vi "Return FPGA Setup Data.vi"(6 "wait for reply (T)":bool=TRUE, 8 "error in (no error)":errorcluster, 10 "Reload":bool) -> (0 "error out":errorcluster, 1 "timed out?":bool, 2 "Reply Payload":T1={"Version String"="", "FPGA Setup Parameters"={"FPGA Timing Constraints"={"frame.length Min"=530, "frame.ST_OFF Min"=15, "frame.ST_ON Min"=8, "frame.first data idx"=14, "frame.integ Offset"=6, "frame.integ Delay"=3, "frame.ad_latch Delay"=11, "frame.trig time Max"=0}, "FPGA Timing Ctrl"={"trig.time"=220, "integ.count 1"=400, "integ.count 2"=350, "encdr.latch ctrl"=1, "pixel.read count"=512, "clock.select"=2, "ad.clock offset"=16, "data.control reg"=2}, "FPGA Laser Config"={"laser.gain"=10, "laser.threshold Low"=1400, "laser.threshold High"=1900, "laser.dac init"=912, "laser.dac Min"=800, "laser.dac Max"=4000, "laser.config reg"=3}, "FPGA Peak Proc Cfg"={"PD.threshold"=0, "PD.width detect Min"=0, "PD.sensor pixels"=512, "PD.config reg"=23}, "FPGA SPI Cfg"={"SPI Divide Value"=1, "SPI config reg"=1}}, "Return FPGA Setup Data_error"={"status"=FALSE, "code"=0, "source"=""}} {"FPGA Setup Parameters"."FPGA SPI Cfg"."SPI config reg" format="%03b"; "FPGA Setup Parameters"."FPGA Peak Proc Cfg"."PD.config reg" format="%05b"; "FPGA Setup Parameters"."FPGA Laser Config"."laser.config reg" format="%02b"; "FPGA Setup Parameters"."FPGA Timing Ctrl"."data.control reg" format="%03b"; "FPGA Setup Parameters"."FPGA Timing Constraints"."frame.trig time Max" format="%0.0f"})   [LabVIEW 2015, in "Tool Module.lvlib"]
doc: "Returns local copy of FPGA setup data from Tool Module.\n_____\nCreated using Delacor QMH Event Scripter 4.2.1.88."
uses:
  Tool Module.lvlib
  Return FPGA Setup Data (Reply Payload)--cluster.ctl
  Tool Typedefs/_FPGA Setup Params Cluster--typedef.ctl
  Tool Typedefs/_FPGA Timing Constraints Cluster--typedef.ctl
  Tool Typedefs/_FPGA Timing Ctrl Cluster--typedef.ctl
  Tool Typedefs/_FPGA Laser Config Cluster--typedef.ctl
  Tool Typedefs/_FPGA Peak Proc Cfg Cluster--typedef.ctl
  Tool Typedefs/_FPGA SPI Cfg Cluster--typedef.ctl
  Return FPGA Setup Data Argument--cluster.ctl
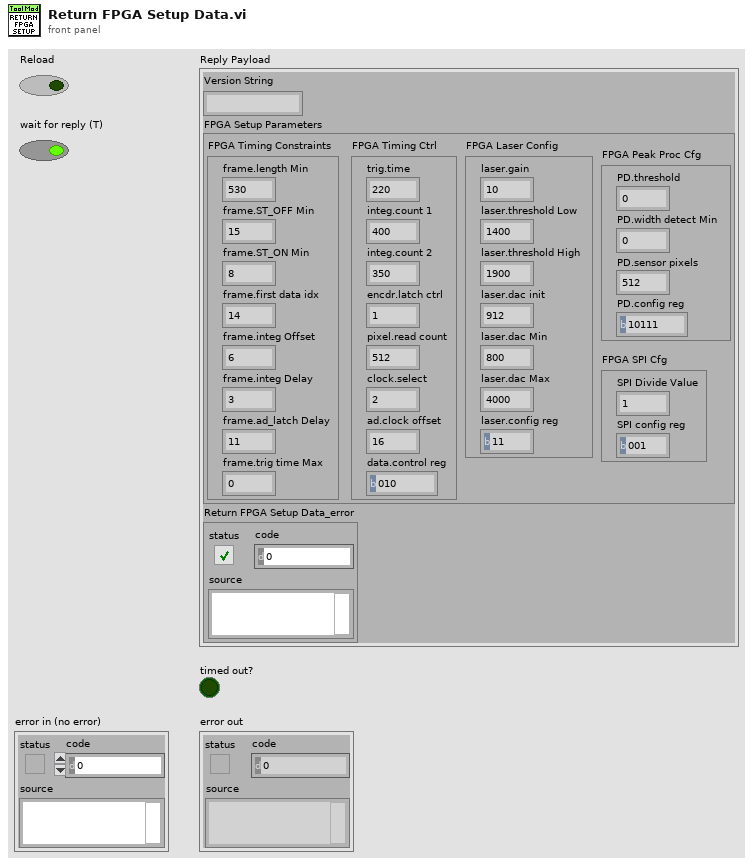
[diagram p1: front panel]
types:
  T1 = typedef "Tool Module.lvlib/Return FPGA Setup Data (Reply Payload)--cluster.ctl" = cluster{"Version String":string, "FPGA Setup Parameters":T2, "Return FPGA Setup Data_error":errorcluster}
  T2 = typedef "_FPGA Setup Params Cluster--typedef.ctl" = cluster{"FPGA Timing Constraints":T3, "FPGA Timing Ctrl":T4, "FPGA Laser Config":T5, "FPGA Peak Proc Cfg":T6, "FPGA SPI Cfg":T7}
  T3 = typedef "_FPGA Timing Constraints Cluster--typedef.ctl" = cluster{"frame.length Min":u16, "frame.ST_OFF Min":u16, "frame.ST_ON Min":u16, "frame.first data idx":u16, "frame.integ Offset":u16, "frame.integ Delay":u16, "frame.ad_latch Delay":u16, "frame.trig time Max":u32}
  T4 = typedef "_FPGA Timing Ctrl Cluster--typedef.ctl" = cluster{"trig.time":u32, "integ.count 1":u32, "integ.count 2":u32, "encdr.latch ctrl":u32, "pixel.read count":u16, "clock.select":u16, "ad.clock offset":u16, "data.control reg":u16}
  T5 = typedef "_FPGA Laser Config Cluster--typedef.ctl" = cluster{"laser.gain":i16, "laser.threshold Low":u16, "laser.threshold High":u16, "laser.dac init":u16, "laser.dac Min":u16, "laser.dac Max":u16, "laser.config reg":u16}
  T6 = typedef "_FPGA Peak Proc Cfg Cluster--typedef.ctl" = cluster{"PD.threshold":u16, "PD.width detect Min":u8, "PD.sensor pixels":u16, "PD.config reg":u16}
  T7 = typedef "_FPGA SPI Cfg Cluster--typedef.ctl" = cluster{"SPI Divide Value":u8, "SPI config reg":u16}
  T8 = typedef "Tool Module.lvlib/Return FPGA Setup Data Argument--cluster.ctl" = cluster{"Reload":bool, "Wait Notifier":refnum<notifier>, "wait for reply":bool}
  T9 = typedef "Tool Module.lvlib/Request Events--cluster.ctl" = cluster{"Stop Module":refnum<user-event>, "Show Panel":refnum<user-event>, "Hide Panel":refnum<user-event>, "Get Module Execution Status":refnum<user-event>, "Show Diagram":refnum<user-event>, "Test Trig 2":refnum<user-event>, "GOTO":refnum<user-event>, "Start Inspect":refnum<user-event>, "CONNECT":refnum<user-event>, "Get All Inspect Data":refnum<user-event>, "Get Inspection Limits":refnum<user-event>, "Set Inspection Limits":refnum<user-event>, "Update Status":refnum<user-event>, "Start Data Monitor":refnum<user-event>, "Get FPGA Setup Params":refnum<user-event>, "Set FPGA Setup Params":refnum<user-event>, "Set Tool Config":refnum<user-event>, "Get Tool Config":refnum<user-event>, "Set Integration Count":refnum<user-event>, "Set Laser Params":refnum<user-event>, "Get Mtrl Ctrl Reg":refnum<user-event>, "Commit Ctrl Reg":refnum<user-event>, "Set Event Logger":refnum<user-event>, "Write to File":refnum<user-event>, "Read from File":refnum<user-event>, "Set Device Temp Thresholds":refnum<user-event>, "Get Cycle Count":refnum<user-event>, "Return FPGA Setup Data":refnum<user-event>, "Update FPGA Setup Data":refnum<user-event>}
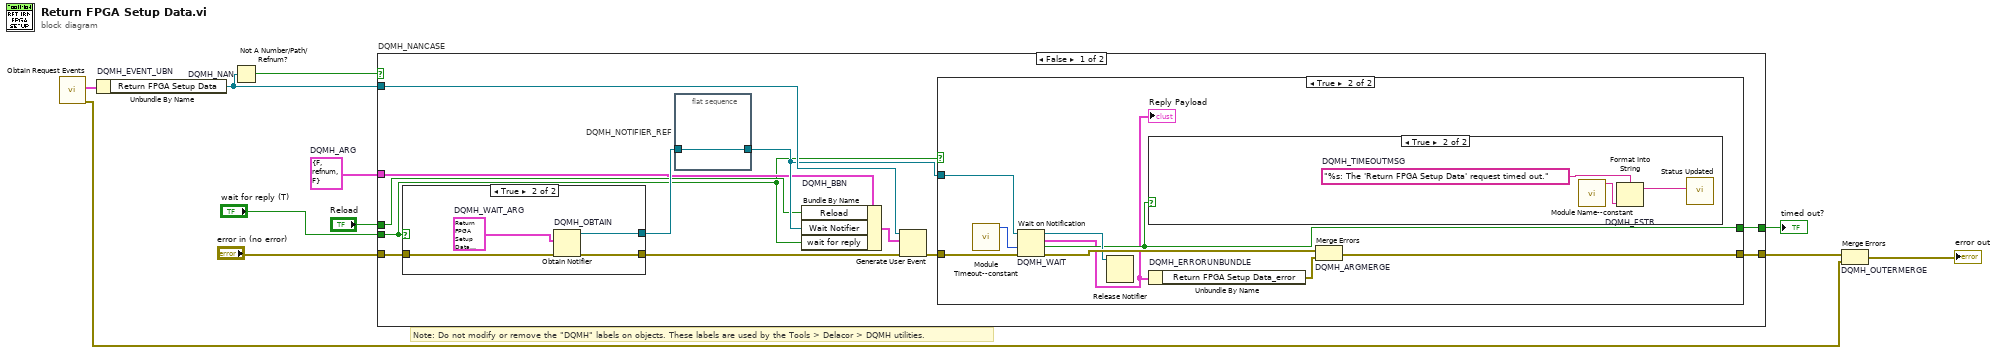
[diagram p0: block diagram]
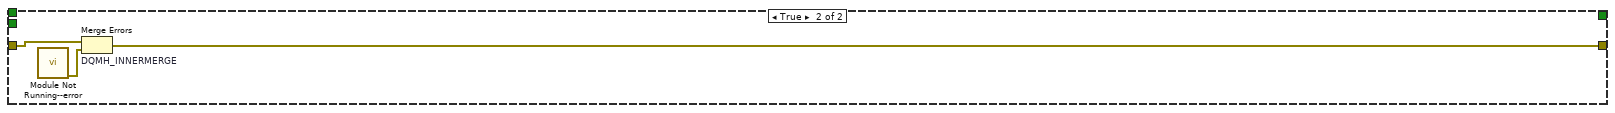
[diagram p5: hidden frame]
diagram:
  w5 = T8 {"Reload"=FALSE, "Wait Notifier"=refnum, "wait for reply"=FALSE}  # DQMH_ARG
  # "Note: Do not modify or remove the \"DQMH\" labels on objects. These labels are used by the Tools > Delacor > DQMH utilities."
  n1 = call "Obtain Request Events.vi"() -> ("error out"=w2:errorcluster, "Tool Module Request Events"=w1:T9)  [unwired: 10 in]
  n2 = Unbundle By Name "DQMH_EVENT_UBN"(w1) -> ("Return FPGA Setup Data"=w9:refnum<user-event>)
  n3 = Not A Number/Path/Refnum? "DQMH_NAN"(number/path/refnum=w9) -> (NaN/Path/Refnum?=w8:bool)
  n4 = case "DQMH_NANCASE" shown="False" w8 {
    tunnel: "error in (no error)" -> [w23 w45]
    tunnel: w9 -> [w21 _]
    tunnel: [w18 w44] -> w6
    tunnel: [w19 _] -> w7
    tunnel: w5 -> [w14 _]
    tunnel: "Reload" -> [w13 _]
    tunnel: "wait for reply (T)" -> [w12 _]
    frame False {
      n5 = case shown="True" w12 {
        tunnel: w23 -> [w38 w42]
        tunnel: [w38 w41] -> w20
        tunnel: [_ w39] -> w16
        frame False {
        }
        frame True {
          w40 = T1 {"Version String"="", "FPGA Setup Parameters"={"FPGA Timing Constraints"={"frame.length Min"=530, "frame.ST_OFF Min"=15, "frame.ST_ON Min"=8, "frame.first data idx"=14, "frame.integ Offset"=6, "frame.integ Delay"=3, "frame.ad_latch Delay"=11, "frame.trig time Max"=0}, "FPGA Timing Ctrl"={"trig.time"=220, "integ.count 1"=400, "integ.count 2"=350, "encdr.latch ctrl"=1, "pixel.read count"=512, "clock.select"=2, "ad.clock offset"=16, "data.control reg"=2}, "FPGA Laser Config"={"laser.gain"=10, "laser.threshold Low"=1400, "laser.threshold High"=1900, "laser.dac init"=912, "laser.dac Min"=800, "laser.dac Max"=4000, "laser.config reg"=3}, "FPGA Peak Proc Cfg"={"PD.threshold"=0, "PD.width detect Min"=0, "PD.sensor pixels"=512, "PD.config reg"=23}, "FPGA SPI Cfg"={"SPI Divide Value"=1, "SPI config reg"=1}}, "Return FPGA Setup Data_error"={"status"=FALSE, "code"=0, "source"=""}}  # DQMH_WAIT_ARG
          n6 = Obtain Notifier "DQMH_OBTAIN"(notification data type=w40, error in (no error)=w42) -> (notifier out=w39:refnum<notifier>, error out=w41:errorcluster)  [unwired: 2 in, 1 out]
        }
      }
      n7 = flat-sequence "DQMH_NOTIFIER_REF" {
        tunnel: w16 -> [w24]
        tunnel: [w24] -> w15
        frame #0 {
        }
      }
      n8 = Bundle By Name "DQMH_BBN"(cluster=w14, "Reload"=w13, "Wait Notifier"=w15, "wait for reply"=w12) -> (w17:T8)
      n9 = Generate User Event(user event=w21, event data cluster=w17, error in=w20) -> (error out=w22:errorcluster)  [unwired: 1 in, 1 out]
      n10 = case shown="True" w12 {
        tunnel: w22 -> [w25 w34]
        tunnel: w15 -> [_ w32]
        tunnel: [_ w30] -> w19
        tunnel: [w25 w29] -> w18
        frame False {
        }
        frame True {
          n11 = call "Module Timeout--constant.vi"() -> ("Module Timeout"=w26:i32)  [unwired: 11 in]
          n12 = Wait on Notification "DQMH_WAIT"(notifier=w32, timeout in ms (-1)=w26, error in (no error)=w34) -> (notifier out=w31:refnum<notifier>, notification=w27:T1, timed out?=w30:bool, error out=w33:errorcluster)  [unwired: 1 in]
          "Reply Payload" <- w27
          n13 = Release Notifier(notifier=w31) -> ()  [unwired: 2 in, 3 out]
          n14 = case shown="True" w30 {
            frame False {
            }
            frame True {
              w37 = "%s: The 'Return FPGA Setup Data' request timed out."  # DQMH_TIMEOUTMSG
              n15 = call "Module Name--constant.vi"() -> ("Module Name"=w36:string)  [unwired: 11 in]
              n16 = Format Into String "DQMH_FSTR"(format string=w37, w36) -> (resulting string=w35:string)  [unwired: 2 in, 1 out]
              n17 = call "Status Updated.vi"("Status"=w35) -> ()  [unwired: 10 in, 1 out]
            }
          }
          n18 = Unbundle By Name "DQMH_ERRORUNBUNDLE"(w27) -> ("Return FPGA Setup Data_error"=w28:errorcluster)
          n19 = Merge Errors "DQMH_ARGMERGE"(w33, w28) -> (w29:errorcluster)
        }
      }
    }
    frame True {
      n20 = call "Module Not Running--error.vi"() -> ("error out"=w43:errorcluster)  [unwired: 11 in]
      n21 = Merge Errors "DQMH_INNERMERGE"(w45, w43) -> (w44:errorcluster)
    }
  }
  "timed out?" <- w7
  n22 = Merge Errors "DQMH_OUTERMERGE"(w6, w2) -> (→"error out":errorcluster)
